vi "CRYGraph Property Window Intensity.vi"(9 "Tab Name":string, 10 "Graph VI Ref":refnum<vi>) -> ()   [LabVIEW 2013]
uses:
  Control/CRYIntensity Property.ctl
panel:
  out "CursorLineStyle":string
  out "CursorLineWidth":string
  out "CursorPointStyle":string
  out "CursorStyle":string
  in  "No Data":bool
  in  "Draw":bool
  in  "Intensity Property":T1 {"Type" items=["Rectangle"=0, "Hanning"=1, "Hamming"=2, "Blackman-Harris"=3, "Exact Blackman"=4, "Blackman"=5, "Flat Top"=6, "4 Term B-Harris"=7, "7 Term B-Harris"=8, "Low Sidelobe"=9, "Blackman Nuttall"=11, "Triangle"=30, "Bartlett-Hanning"=31, "Bohman"=32, "Parzen"=33, "Welch"=34, "Kaiser"=60, "Dolph-Chebyshev"=61, "Gaussian"=62]}
  in  "Intensity Tab":enum32{"Title", "Plot", "Cursor"}(tab)
  in  "Background Color":u32(colorbox) caption="aa"
  in  "Title Name":string caption="aa"
  in  "Length":i32=1 caption="aa" min=1 step=1
  in  "Type":u32(ring) caption="aa" items=["Rectangle"=0, "Hanning"=1, "Hamming"=2, "Blackman-Harris"=3, "Exact Blackman"=4, "Blackman"=5, "Flat Top"=6, "4 Term B-Harris"=7, "7 Term B-Harris"=8, "Low Sidelobe"=9, "Blackman Nuttall"=11, "Triangle"=30, "Bartlett-Hanning"=31, "Bohman"=32, "Parzen"=33, "Welch"=34, "Kaiser"=60, "Dolph-Chebyshev"=61, "Gaussian"=62]
  out "Window":bool caption="aa"
  in  "Frequency Bins":i32=1 caption="aa间隔" min=1 step=1
  in  "Time Steps":i32=1 caption="aa" min=1 step=1
  out "Time-Freq Sampling":bool caption="aa"
  in  "ColorMap Type":u16(ring) caption="aa" items=["Fire", "Rainbow", "Log up", "Log down", "Colour", "Ice"]
  in  "Show Cursors":bool caption="aa"
  in  "Cursor Tab":enum32{"Page 1"}(tab)
  in  "CursorPointStyle16":bool
  in  "CursorPointStyle15":bool
  in  "CursorPointStyle14":bool
  in  "CursorPointStyle13":bool
  in  "CursorPointStyle12":bool
  in  "CursorPointStyle11":bool
  in  "CursorPointStyle10":bool
  in  "CursorPointStyle9":bool
  in  "CursorPointStyle8":bool
  in  "CursorPointStyle7":bool
  in  "CursorPointStyle6":bool
  in  "CursorPointStyle5":bool
  in  "CursorPointStyle4":bool
  in  "CursorPointStyle3":bool
  in  "CursorPointStyle2":bool
  in  "CursorPointStyle1":bool
  in  "CursorPointStyle0":bool
  in  "CursorLineWidth5":bool
  in  "CursorLineWidth1":bool
  in  "CursorLineWidth4":bool
  in  "CursorLineWidth3":bool
  in  "CursorLineWidth2":bool
  in  "CursorLineWidth0":bool
  in  "CursorLineStyle4":bool
  in  "CursorLineStyle3":bool
  in  "CursorLineStyle2":bool
  in  "CursorLineStyle0":bool
  in  "CursorLineStyle1":bool
  in  "Cursor Items":u16(ring)
  in  "CursorStyle8":bool
  in  "CursorStyle4":bool
  in  "CursorStyle5":bool
  in  "CursorStyle7":bool
  in  "CursorStyle6":bool
  in  "CursorStyle3":bool
  in  "CursorStyle2":bool
  in  "CursorStyle1":bool
  in  "CursorStyle0":bool
  in  "Cursor color":u32(colorbox) caption="aa"
  in  "OK":bool
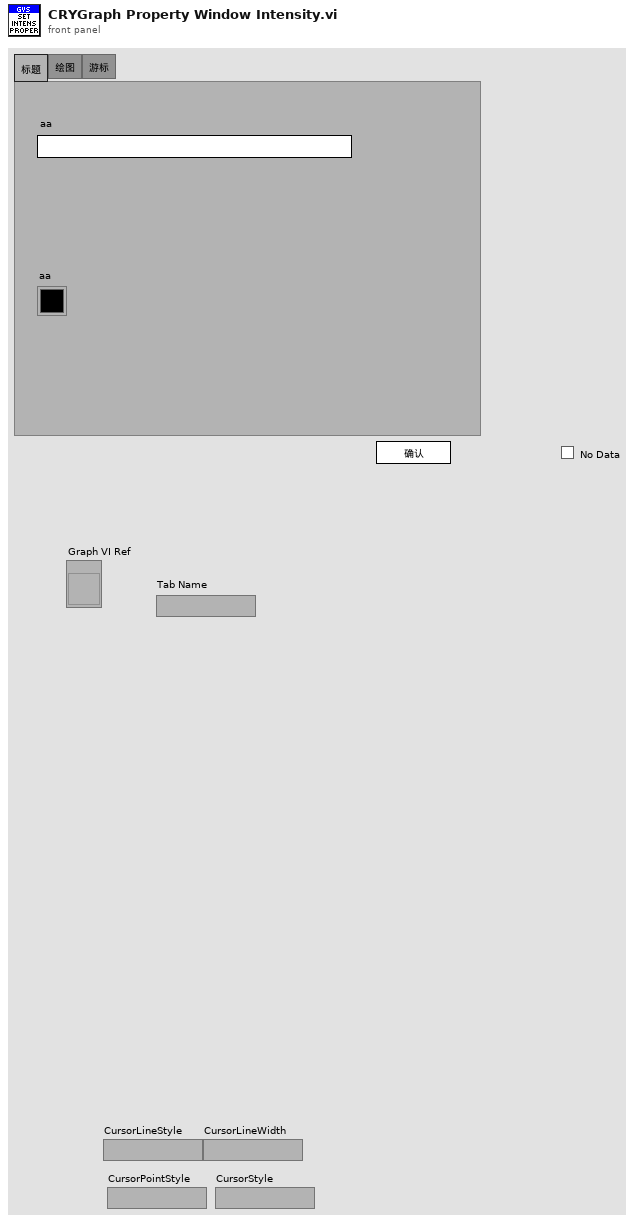
[diagram p1: front panel]
types:
  T1 = typedef "CRYIntensity Property.ctl" = cluster{"Time Steps":i32, "Frequency Bins":i32, "Type":u32, "Length":i32, "Map Type":enum16{"fire", "rainbow", "grey", "inverse grey", "ice", "original"}}
  T2 = enum32{"Page Enabled", "Page Disabled", "Page Disabled & Grayed"}
  T3 = enum16{"fire", "rainbow", "grey", "inverse grey", "ice", "original"}
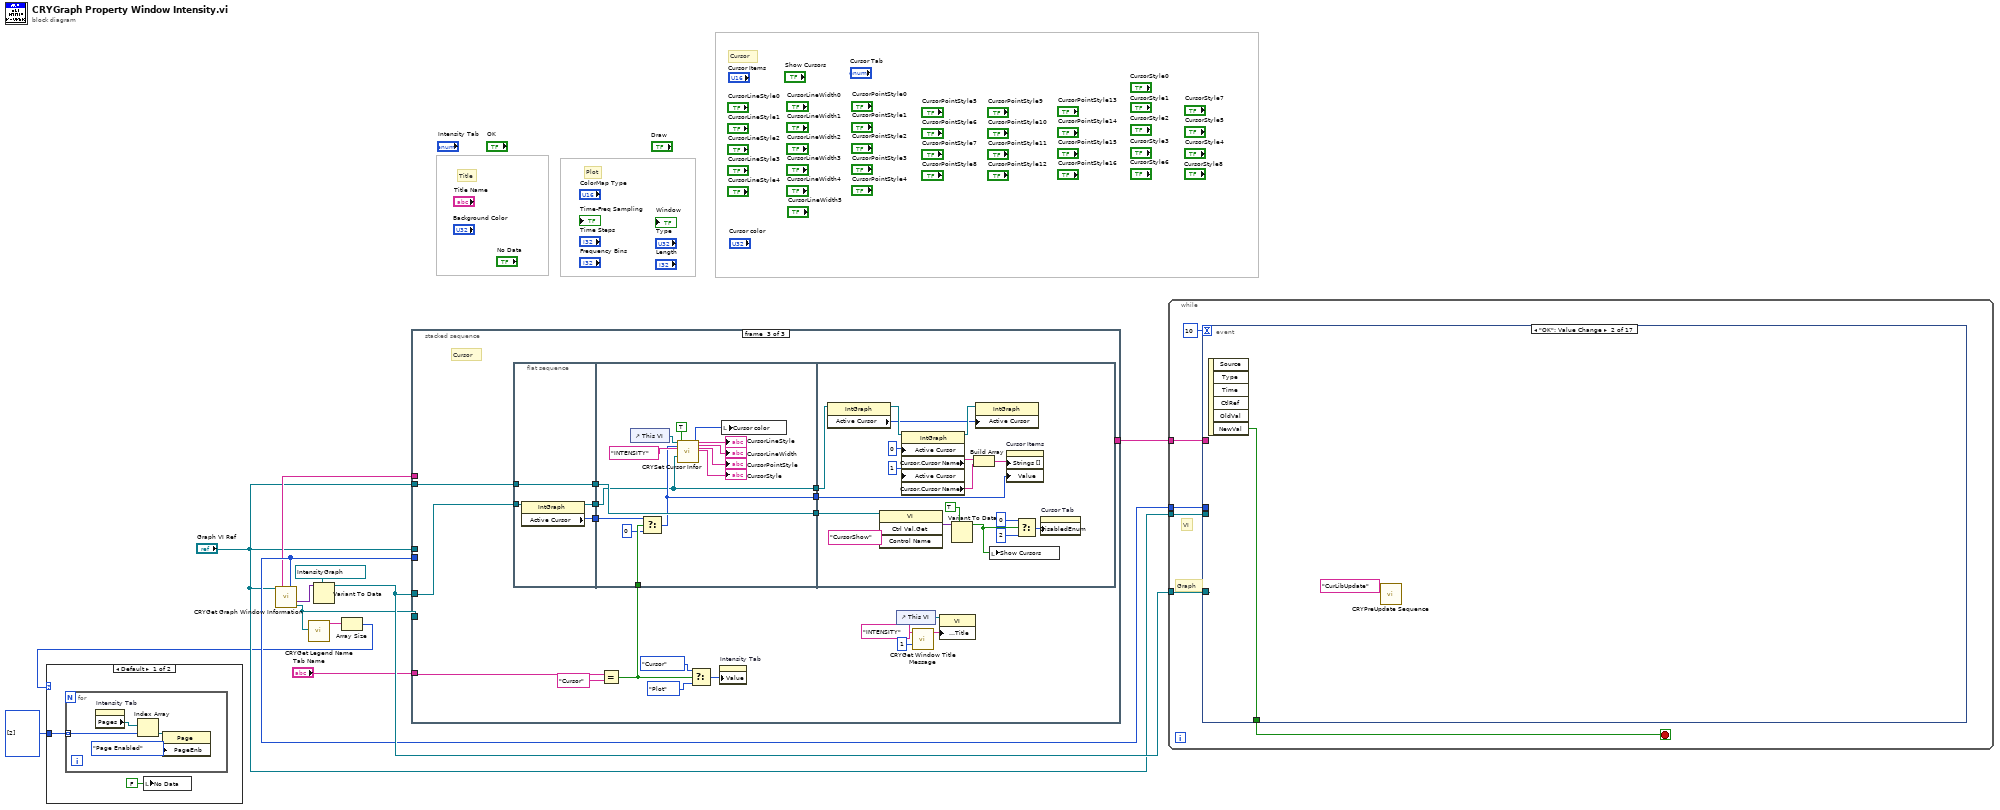
[diagram p0: block diagram]
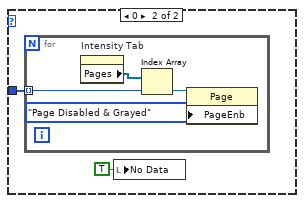
[diagram p2: hidden frame]
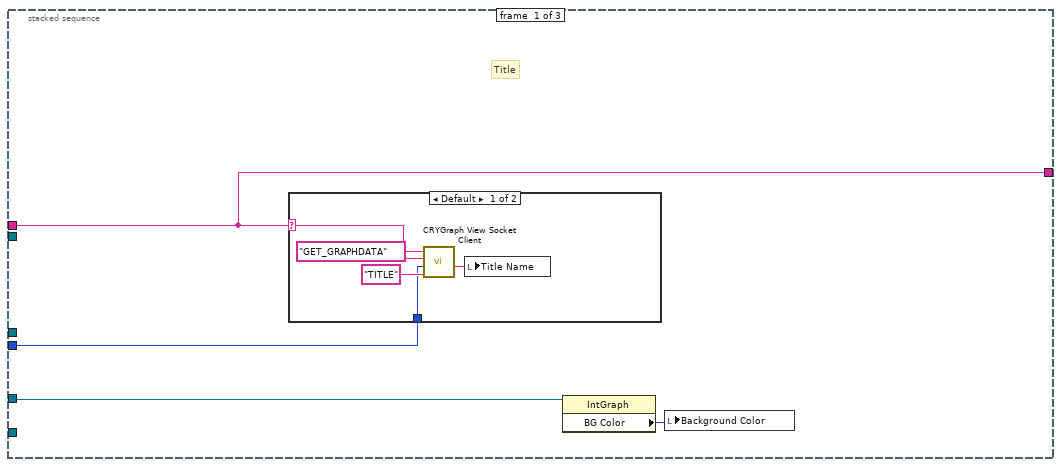
[diagram p3: hidden frame]
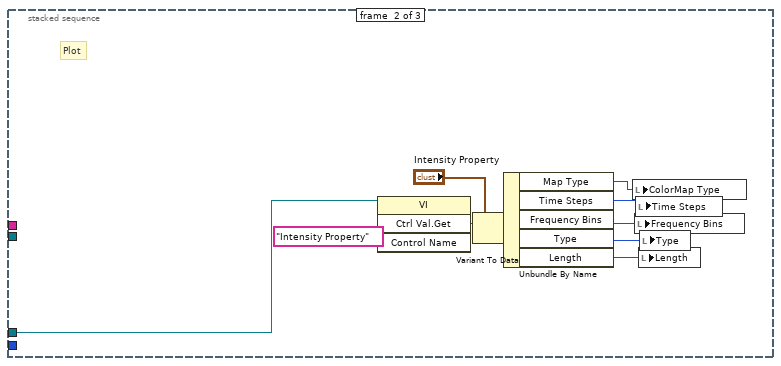
[diagram p5: hidden frame]
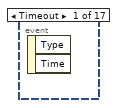
[diagram p6: hidden frame]
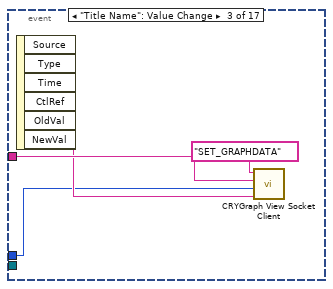
[diagram p7: hidden frame]
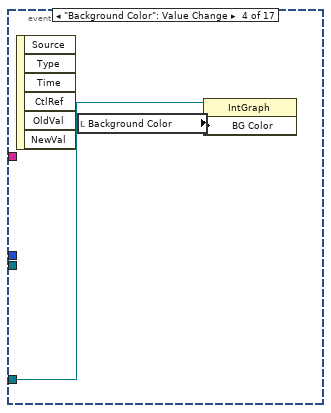
[diagram p8: hidden frame]
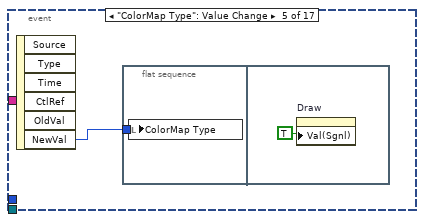
[diagram p9: hidden frame]
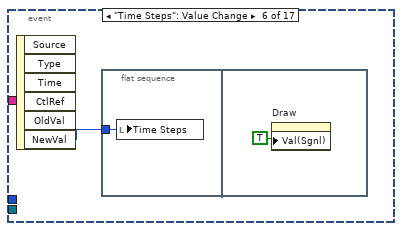
[diagram p10: hidden frame]
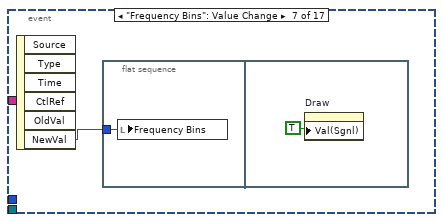
[diagram p11: hidden frame]
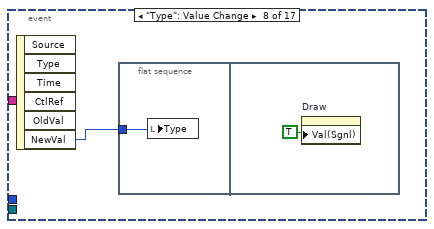
[diagram p12: hidden frame]
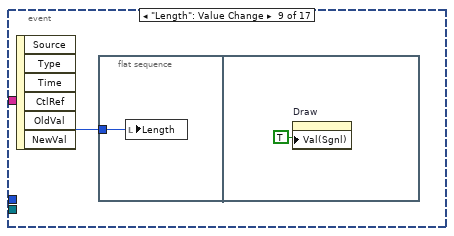
[diagram p13: hidden frame]
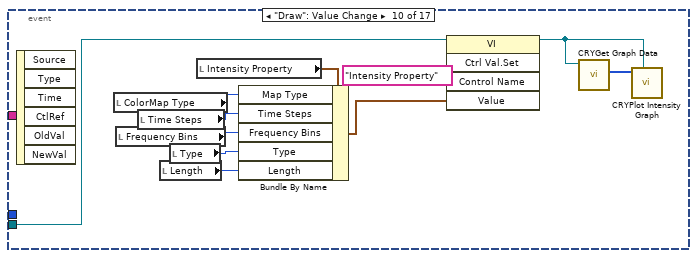
[diagram p14: hidden frame]
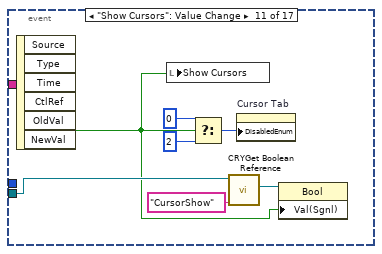
[diagram p15: hidden frame]
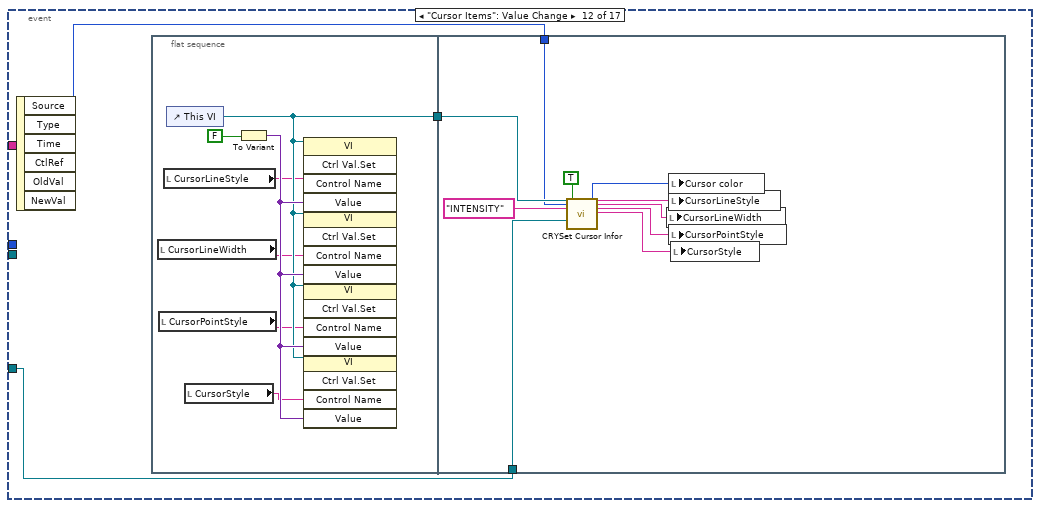
[diagram p16: hidden frame]
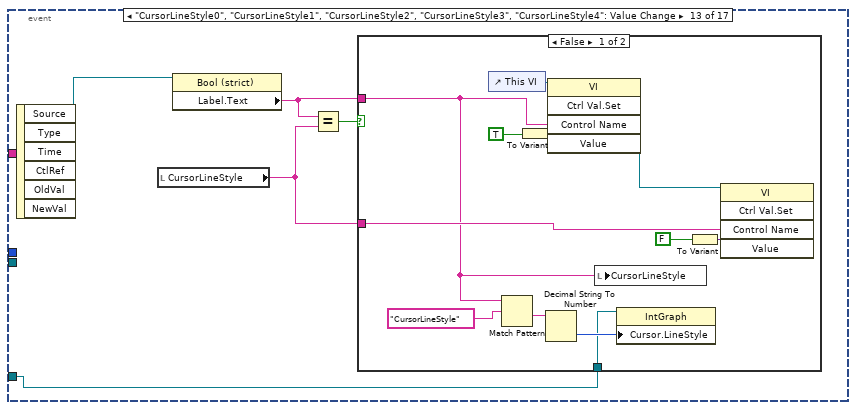
[diagram p17: hidden frame]
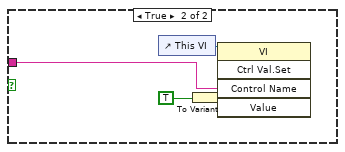
[diagram p18: hidden frame]
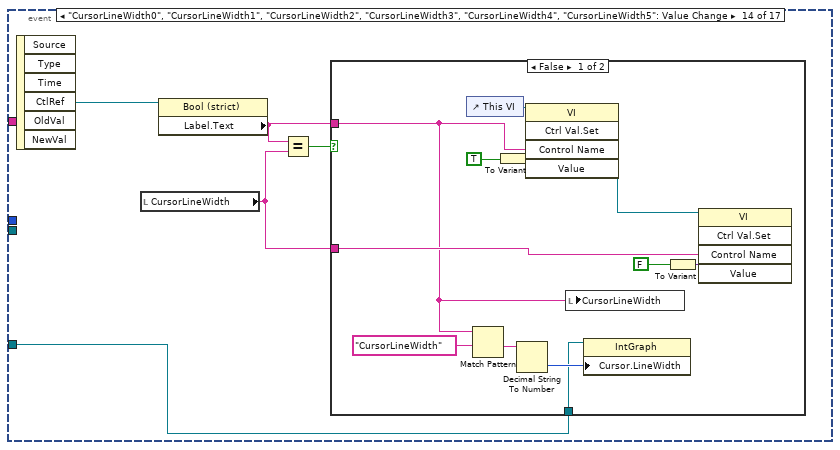
[diagram p19: hidden frame]
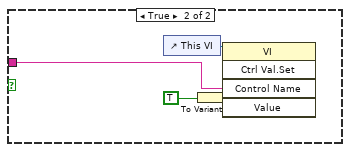
[diagram p20: hidden frame]
diagram:
  # "Cursor"
  # "Title"
  # "Plot"
  n1 = call "CRYGet Graph Window Information.vi"("pGraph VI In"="Graph VI Ref") -> ("Queue Name Out"=w10:string, "Graph Number Out"=w11:i32, "Graph Control Ref Out"=w4:variant, "Legend Ref Out"=w7:refnum<vi>)  [unwired: 4 in, 7 out]
  n2 = call "CRYGet Legend Name.vi"("MCListbox Refnum"=w7) -> ("Names Out"=w2:string[])  [unwired: 1 in, 9 out]
  n3 = Variant To Data(type=refnum<vi> refnum ("Graph Ref"), Variant=w4) -> (data=w12:refnum<vi>)  [unwired: 1 in, 1 out]
  n4 = Array Size(array=w2) -> (size(s)=w1:i32)
  n5 = case shown="Default" w1 {
    tunnel: i32[] [2] -> [w13 w19]
    frame Default {
      n6 = for {
        tunnel: w13 -> [w16] mode=indexing
        n7 = property on="Intensity Tab" class="TabCtl (strict)"() -> ("Pages"=w15:refnum<vi>[])  [unwired: 2 in, 2 out]
        n8 = Index Array(array=w15, index=w16) -> (element=w17:refnum<vi>)
        n9 = property class="Page"(reference=w17, "PageEnb"=T2."Page Enabled" ("Page Enabled State")) -> ()  [unwired: 1 in, 2 out]
      }
      n10 = local write "No Data"(FALSE ("No Data")) -> ()
    }
    frame 0 {
      n11 = for {
        tunnel: w19 -> [w21] mode=indexing
        n12 = property on="Intensity Tab" class="TabCtl (strict)"() -> ("Pages"=w22:refnum<vi>[])  [unwired: 2 in, 2 out]
        n13 = Index Array(array=w22, index=w21) -> (element=w23:refnum<vi>)
        n14 = property class="Page"(reference=w23, "PageEnb"=T2."Page Disabled & Grayed" ("Page Enabled State")) -> ()  [unwired: 1 in, 2 out]
      }
      n15 = local write "No Data"(TRUE ("No Data")) -> ()
    }
  }
  n16 = stacked-sequence {
    tunnel: w12 -> [w27 _ w49]
    tunnel: w11 -> [w26 _ _]
    tunnel: w7 -> [_ _ _]
    tunnel: "Graph VI Ref" -> [_ w41 _]
    tunnel: w10 -> [w25 _ _]
    tunnel: [w25 _ _] -> w9
    tunnel: "Tab Name" -> [_ _ w45]
    tunnel: "Graph VI Ref" -> [_ _ w48]
    frame #0 {
      # "Title"
      n17 = case shown="Default" w25 {
        selector: w25 -> [w30 _]
        tunnel: w26 -> [w31 _]
        frame Default {
          n18 = call "CRYGraph View Socket Client.vi"("sOption"="TITLE", "nData"=w31, "sData"=w30, "sAction"="GET_GRAPHDATA") -> ("sData Out"=w29:string)  [unwired: 4 in, 3 out]
          n19 = local write "Title Name"(w29) -> ()
        }
        frame "test DataView" {
        }
      }
      n20 = property class="IntGraph"(reference=w27) -> ("BG Color"=w28:u32)  [unwired: 1 in, 2 out]
      n21 = local write "Background Color"(w28) -> ()
    }
    frame #1 {
      # "Plot"
      n22 = invoke class="VI" method="Ctrl Val.Get"(reference=w41, "Control Name"="Intensity Property") -> ("Get Control Value Variant"=w42:variant)  [unwired: 2 in, 3 out]
      n23 = Variant To Data(type="Intensity Property", Variant=w42) -> (data=w39:T1)  [unwired: 1 in, 1 out]
      n24 = Unbundle By Name(w39) -> ("Map Type"=w38:T3, "Time Steps"=w37:i32, "Frequency Bins"=w36:i32, "Type"=w35:u32, "Length"=w34:i32)
      n25 = local write "ColorMap Type"(w38) -> ()
      n26 = local write "Frequency Bins"(w36) -> ()
      n27 = local write "Time Steps"(w37) -> ()
      n28 = local write "Length"(w34) -> ()
      n29 = local write "Type"(w35) -> ()
    }
    frame #2 {
      # "Cursor"
      n30 = flat-sequence {
        tunnel: w48 -> [w65]
        tunnel: w49 -> [w64]
        tunnel: [w63] -> w61
        tunnel: [w65] -> w60
        tunnel: [w62] -> w59
        tunnel: [w66] -> w58
        tunnel: [w71] -> w57
        tunnel: w61 -> [w66]
        tunnel: w60 -> [w71]
        tunnel: w51 -> [w70]
        tunnel: w59 -> [w68]
        tunnel: [w67] -> w56
        tunnel: w58 -> [w84]
        tunnel: w57 -> [w85]
        tunnel: w56 -> [w80]
        frame #0 {
          n31 = property class="IntGraph"(reference=w64) -> (reference out=w63:refnum<vi>, "Active Cursor"=w62:u32)  [unwired: 1 in, 1 out]
        }
        frame #1 {
          n32 = control-ref of="This VI"() -> (w72:refnum<vi>)
          n33 = Select(t=w68, s=w70, f=u32 0 ("Active Cursor")) -> (s? t:f=w67:u32)
          n34 = call "CRYSet Cursor Infor.vi"("This VI"=w72, "Active Cursor"=w67, "Graph Type"="INTENSITY", "Intensity Graph Ref"=w66, "Property Set?"=TRUE) -> ("Cursor Color"=w79:u32, "CursorLineStyle"=→"CursorLineStyle":string, "CursorLineWidth"=→"CursorLineWidth":string, "CursorPointStyle"=→"CursorPointStyle":string, "CursorStyle"=→"CursorStyle":string)  [unwired: 17 in, 1 out]
          n35 = local write "Cursor color"(w79) -> ()
        }
        frame #2 {
          n36 = property class="IntGraph"(reference=w84) -> (reference out=w83:refnum<vi>, "Active Cursor"=w81:u32)  [unwired: 1 in, 1 out]
          n37 = invoke class="VI" method="Ctrl Val.Get"(reference=w85, "Control Name"="CursorShow") -> ("Get Control Value Variant"=w90:variant)  [unwired: 2 in, 3 out]
          n38 = property class="IntGraph"(reference=w83, "Active Cursor"=u32 0, "Active Cursor"=u32 1) -> (reference out=w82:refnum<vi>, "Cursor.Cursor Name"=w95:string, "Cursor.Cursor Name"=w94:string)  [unwired: 1 in, 1 out]
          n39 = Variant To Data(type=TRUE ("Visible"), Variant=w90) -> (data=w92:bool)  [unwired: 1 in, 1 out]
          n40 = Build Array(w95, w94) -> (w93:string[])
          n41 = property class="IntGraph"(reference=w82, "Active Cursor"=w81) -> ()  [unwired: 1 in, 2 out]
          n42 = local write "Show Cursors"(w92) -> ()
          n43 = property on="Cursor Items" class="Ring (strict)"("Strings []"=w93, "Value"=w80) -> ()  [unwired: 2 in, 2 out]
          n44 = Select(t=0, s=w92, f=2) -> (s? t:f=w88:i32)
          n45 = property on="Cursor Tab" class="TabCtl (strict)"("DisabledEnum"=w88) -> ()  [unwired: 2 in, 2 out]
        }
      }
      n46 = Equal?(x=w45, y="Cursor" ("Graph Type")) -> (x = y?=w51:bool)
      n47 = Select(t=enum32{"Title", "Plot", "Cursor"}."Cursor" ("Intensity Tab"), s=w51, f=enum32{"Title", "Plot", "Cursor"}."Plot" ("Intensity Tab")) -> (s? t:f=w46:enum32{"Title", "Plot", "Cursor"})
      n48 = property on="Intensity Tab" class="TabCtl (strict)"("Value"=w46) -> ()  [unwired: 2 in, 2 out]
      n49 = control-ref of="This VI"() -> (w55:refnum<vi>)
      n50 = call "CRYGet Window Title Message.vi"("No"=1 ("Error No"), "Kind"="INTENSITY") -> ("Multibyte String"=w54:string)  [unwired: 4 in, 5 out]
      n51 = property class="VI"(reference=w55, "Front Panel.Title"=w54) -> ()  [unwired: 1 in, 2 out]
    }
  }
  n52 = while {
    tunnel: w12 -> [w102]
    tunnel: w11 -> [w101]
    tunnel: "Graph VI Ref" -> [w100]
    tunnel: w9 -> [w99]
    stop <- w103 stop-if-true
    # "Graph"
    # "VI"
    n53 = event shown="[1] \"OK\": Value Change" {
      selector: _ -> [_ _ _ _ _ _ _ _ _ _ _ _ _ _ _ _ _]
      dyn-events: _ -> [_ _ _ _ _ _ _ _ _ _ _ _ _ _ _ _ _]
      timeout: 10 -> [_ _ _ _ _ _ _ _ _ _ _ _ _ _ _ _ _]
      tunnel: [_ w105 _ _ _ _ _ _ _ _ _ _ _ _ _ _ _] -> w103
      tunnel: w102 -> [_ _ _ w111 _ _ _ _ _ _ _ w146 w166 w186 w207 w228 w250]
      tunnel: w101 -> [_ _ w106 _ _ _ _ _ _ _ _ _ _ _ _ _ _]
      tunnel: w100 -> [_ _ _ _ _ _ _ _ _ w137 w139 _ _ _ _ _ w249]
      tunnel: w99 -> [_ _ w108 _ _ _ _ _ _ _ _ _ _ _ _ _ _]
      event Timeout {
        n54 = event-data() -> ()  [unwired: 3 out]
      }
      event "OK": Value Change {
        n55 = event-data() -> ("NewVal"=w105:bool)  [unwired: 6 out]
        n56 = call "CRYPreUpdate Sequence.vi"("EventName"="CurLibUpdate") -> ()  [unwired: 15 in]
      }
      event "Title Name": Value Change {
        n57 = event-data() -> ("NewVal"=w107:string)  [unwired: 6 out]
        n58 = call "CRYGraph View Socket Client.vi"("sOption"=w107, "nData"=w106, "sData"=w108, "sAction"="SET_GRAPHDATA") -> ()  [unwired: 4 in, 4 out]
      }
      event "Background Color": Value Change {
        n59 = event-data() -> ()  [unwired: 7 out]
        n60 = local read "Background Color"() -> (w110:u32)
        n61 = property class="IntGraph"(reference=w111, "BG Color"=w110) -> ()  [unwired: 1 in, 2 out]
      }
      event "ColorMap Type": Value Change {
        n62 = event-data() -> ("NewVal"=w112:u16)  [unwired: 6 out]
        n63 = flat-sequence {
          tunnel: w112 -> [w113]
          frame #0 {
            n64 = local write "ColorMap Type"(w113) -> ()
          }
          frame #1 {
            n65 = property on="Draw" class="Bool (strict)"("Val(Sgnl)"=TRUE ("Value (Signaling)")) -> ()  [unwired: 2 in, 2 out]
          }
        }
      }
      event "Time Steps": Value Change {
        n66 = event-data() -> ("NewVal"=w115:i32)  [unwired: 6 out]
        n67 = flat-sequence {
          tunnel: w115 -> [w116]
          frame #0 {
            n68 = local write "Time Steps"(w116) -> ()
          }
          frame #1 {
            n69 = property on="Draw" class="Bool (strict)"("Val(Sgnl)"=TRUE ("Value (Signaling)")) -> ()  [unwired: 2 in, 2 out]
          }
        }
      }
      event "Frequency Bins": Value Change {
        n70 = event-data() -> ("NewVal"=w118:i32)  [unwired: 6 out]
        n71 = flat-sequence {
          tunnel: w118 -> [w119]
          frame #0 {
            n72 = local write "Frequency Bins"(w119) -> ()
          }
          frame #1 {
            n73 = property on="Draw" class="Bool (strict)"("Val(Sgnl)"=TRUE ("Value (Signaling)")) -> ()  [unwired: 2 in, 2 out]
          }
        }
      }
      event "Type": Value Change {
        n74 = event-data() -> ("NewVal"=w121:u32)  [unwired: 6 out]
        n75 = flat-sequence {
          tunnel: w121 -> [w122]
          frame #0 {
            n76 = local write "Type"(w122) -> ()
          }
          frame #1 {
            n77 = property on="Draw" class="Bool (strict)"("Val(Sgnl)"=TRUE ("Value (Signaling)")) -> ()  [unwired: 2 in, 2 out]
          }
        }
      }
      event "Length": Value Change {
        n78 = event-data() -> ("NewVal"=w124:i32)  [unwired: 6 out]
        n79 = flat-sequence {
          tunnel: w124 -> [w125]
          frame #0 {
            n80 = local write "Length"(w125) -> ()
          }
          frame #1 {
            n81 = property on="Draw" class="Bool (strict)"("Val(Sgnl)"=TRUE ("Value (Signaling)")) -> ()  [unwired: 2 in, 2 out]
          }
        }
      }
      event "Draw": Value Change {
        n82 = event-data() -> ()  [unwired: 7 out]
        n83 = local read "ColorMap Type"() -> (w134:u16)
        n84 = local read "Frequency Bins"() -> (w132:i32)
        n85 = local read "Time Steps"() -> (w133:i32)
        n86 = local read "Length"() -> (w130:i32)
        n87 = local read "Type"() -> (w131:u32)
        n88 = local read "Intensity Property"() -> (w135:T1)
        n89 = Bundle By Name(cluster=w135, "Map Type"=w134, "Time Steps"=w133, "Frequency Bins"=w132, "Type"=w131, "Length"=w130) -> (w129:T1)
        n90 = invoke class="VI" method="Ctrl Val.Set"(reference=w137, "Control Name"="Intensity Property", "Value"=w129) -> (reference out=w127:refnum<vi>)  [unwired: 2 in, 4 out]
        n91 = call "CRYGet Graph Data.vi"("pGraph VI"=w127) -> ("Rows"=w128:i32[])  [unwired: 2 in, 8 out]
        n92 = call "CRYPlot Intensity Graph.vi"("pGraph VI In"=w127, "Selected Rows In"=w128) -> ()  [unwired: 6 in, 4 out]
      }
      event "Show Cursors": Value Change {
        n93 = event-data() -> ("NewVal"=w138:bool)  [unwired: 6 out]
        n94 = local write "Show Cursors"(w138) -> ()
        n95 = Select(t=0, s=w138, f=2) -> (s? t:f=w140:i32)
        n96 = call "CRYGet Boolean Reference.vi"("Label Name"="CursorShow", "VI Refnum"=w139) -> ("Boolean Ref"=w144:refnum<vi>)  [unwired: 7 in, 2 out]
        n97 = property on="Cursor Tab" class="TabCtl (strict)"("DisabledEnum"=w140) -> ()  [unwired: 2 in, 2 out]
        n98 = property class="Bool"(reference=w144, "Val(Sgnl)"=w138) -> ()  [unwired: 1 in, 2 out]
      }
      event "Cursor Items": Value Change {
        n99 = event-data() -> ("NewVal"=w145:u16)  [unwired: 6 out]
        n100 = flat-sequence {
          tunnel: [w152] -> w147
          tunnel: w147 -> [w157]
          tunnel: w145 -> [w156]
          tunnel: w146 -> [w155]
          frame #0 {
            n101 = local read "CursorLineWidth"() -> (w150:string)
            n102 = local read "CursorPointStyle"() -> (w149:string)
            n103 = local read "CursorLineStyle"() -> (w151:string)
            n104 = control-ref of="This VI"() -> (w152:refnum<vi>)
            n105 = local read "CursorStyle"() -> (w148:string)
            n106 = To Variant(anything=FALSE) -> (Variant=w154:variant)
            n107 = invoke class="VI" method="Ctrl Val.Set"(reference=w152, "Control Name"=w151, "Value"=w154) -> ()  [unwired: 2 in, 5 out]
            n108 = invoke class="VI" method="Ctrl Val.Set"(reference=w152, "Control Name"=w150, "Value"=w154) -> ()  [unwired: 2 in, 5 out]
            n109 = invoke class="VI" method="Ctrl Val.Set"(reference=w152, "Control Name"=w149, "Value"=w154) -> ()  [unwired: 2 in, 5 out]
            n110 = invoke class="VI" method="Ctrl Val.Set"(reference=w152, "Control Name"=w148, "Value"=w154) -> ()  [unwired: 2 in, 5 out]
          }
          frame #1 {
            n111 = call "CRYSet Cursor Infor.vi"("This VI"=w157, "Active Cursor"=w156, "Graph Type"="INTENSITY", "Intensity Graph Ref"=w155, "Property Set?"=TRUE) -> ("Cursor Color"=w158:u32, "CursorLineStyle"=w161:string, "CursorLineWidth"=w162:string, "CursorPointStyle"=w163:string, "CursorStyle"=w164:string)  [unwired: 17 in, 1 out]
            n112 = local write "CursorLineWidth"(w162) -> ()
            n113 = local write "Cursor color"(w158) -> ()
            n114 = local write "CursorLineStyle"(w161) -> ()
            n115 = local write "CursorPointStyle"(w163) -> ()
            n116 = local write "CursorStyle"(w164) -> ()
          }
        }
      }
      event "CursorLineStyle0", "CursorLineStyle1", "CursorLineStyle2", "CursorLineStyle3", "CursorLineStyle4": Value Change {
        n117 = event-data() -> ("CtlRef"=w165:refnum<vi>)  [unwired: 6 out]
        n118 = local read "CursorLineStyle"() -> (w169:string)
        n119 = property class="Bool (strict)"(reference=w165) -> ("Label.Text"=w167:string)  [unwired: 1 in, 2 out]
        n120 = Equal?(x=w167, y=w169) -> (x = y?=w168:bool)
        n121 = case shown="False" w168 {
          tunnel: w167 -> [w170 w182]
          tunnel: w169 -> [w180 _]
          tunnel: w166 -> [w171 _]
          frame False {
            n122 = control-ref of="This VI"() -> (w181:refnum<vi>)
            n123 = Match Pattern(string=w170, regular expression="CursorLineStyle") -> (after substring=w173:string)  [unwired: 4 out]
            n124 = To Variant(anything=TRUE) -> (Variant=w178:variant)
            n125 = Decimal String To Number(string=w173) -> (number=w172:i32)  [unwired: 3 out]
            n126 = invoke class="VI" method="Ctrl Val.Set"(reference=w181, "Control Name"=w170, "Value"=w178) -> (reference out=w179:refnum<vi>)  [unwired: 2 in, 4 out]
            n127 = local write "CursorLineStyle"(w170) -> ()
            n128 = property class="IntGraph"(reference=w171, "Cursor.LineStyle"=w172) -> ()  [unwired: 1 in, 2 out]
            n129 = To Variant(anything=FALSE) -> (Variant=w176:variant)
            n130 = invoke class="VI" method="Ctrl Val.Set"(reference=w179, "Control Name"=w180, "Value"=w176) -> ()  [unwired: 2 in, 5 out]
          }
          frame True {
            n131 = control-ref of="This VI"() -> (w185:refnum<vi>)
            n132 = To Variant(anything=TRUE) -> (Variant=w184:variant)
            n133 = invoke class="VI" method="Ctrl Val.Set"(reference=w185, "Control Name"=w182, "Value"=w184) -> ()  [unwired: 2 in, 5 out]
          }
        }
      }
      event "CursorLineWidth0", "CursorLineWidth1", "CursorLineWidth2", "CursorLineWidth3", "CursorLineWidth4", "CursorLineWidth5": Value Change {
        n134 = event-data() -> ("CtlRef"=w187:refnum<vi>)  [unwired: 6 out]
        n135 = local read "CursorLineWidth"() -> (w190:string)
        n136 = property class="Bool (strict)"(reference=w187) -> ("Label.Text"=w188:string)  [unwired: 1 in, 2 out]
        n137 = Equal?(x=w188, y=w190) -> (x = y?=w189:bool)
        n138 = case shown="False" w189 {
          tunnel: w188 -> [w191 w203]
          tunnel: w190 -> [w201 _]
          tunnel: w186 -> [w192 _]
          frame False {
            n139 = control-ref of="This VI"() -> (w202:refnum<vi>)
            n140 = Match Pattern(string=w191, regular expression="CursorLineWidth") -> (after substring=w194:string)  [unwired: 4 out]
            n141 = To Variant(anything=TRUE) -> (Variant=w199:variant)
            n142 = Decimal String To Number(string=w194) -> (number=w195:i32)  [unwired: 3 out]
            n143 = invoke class="VI" method="Ctrl Val.Set"(reference=w202, "Control Name"=w191, "Value"=w199) -> (reference out=w200:refnum<vi>)  [unwired: 2 in, 4 out]
            n144 = local write "CursorLineWidth"(w191) -> ()
            n145 = property class="IntGraph"(reference=w192, "Cursor.LineWidth"=w195) -> ()  [unwired: 1 in, 2 out]
            n146 = To Variant(anything=FALSE) -> (Variant=w197:variant)
            n147 = invoke class="VI" method="Ctrl Val.Set"(reference=w200, "Control Name"=w201, "Value"=w197) -> ()  [unwired: 2 in, 5 out]
          }
          frame True {
            n148 = control-ref of="This VI"() -> (w206:refnum<vi>)
            n149 = To Variant(anything=TRUE) -> (Variant=w205:variant)
            n150 = invoke class="VI" method="Ctrl Val.Set"(reference=w206, "Control Name"=w203, "Value"=w205) -> ()  [unwired: 2 in, 5 out]
          }
        }
      }
      event "CursorPointStyle0", "CursorPointStyle1", "CursorPointStyle2", "CursorPointStyle3", "CursorPointStyle4", "CursorPointStyle5", "CursorPointStyle6", "CursorPointStyle7", "CursorPointStyle8", "CursorPointStyle9", "CursorPointStyle10", "CursorPointStyle11", "CursorPointStyle12", "CursorPointStyle13", "CursorPointStyle14", "CursorPointStyle15", "CursorPointStyle16": Value Change {
        n151 = event-data() -> ("CtlRef"=w208:refnum<vi>)  [unwired: 6 out]
        n152 = local read "CursorPointStyle"() -> (w211:string)
        n153 = property class="Bool (strict)"(reference=w208) -> ("Label.Text"=w209:string)  [unwired: 1 in, 2 out]
        n154 = Equal?(x=w209, y=w211) -> (x = y?=w210:bool)
        n155 = case shown="False" w210 {
          tunnel: w209 -> [w212 w224]
          tunnel: w211 -> [w222 _]
          tunnel: w207 -> [w213 _]
          frame False {
            n156 = control-ref of="This VI"() -> (w223:refnum<vi>)
            n157 = To Variant(anything=TRUE) -> (Variant=w220:variant)
            n158 = Match Pattern(string=w212, regular expression="CursorPointStyle") -> (after substring=w215:string)  [unwired: 4 out]
            n159 = invoke class="VI" method="Ctrl Val.Set"(reference=w223, "Control Name"=w212, "Value"=w220) -> (reference out=w221:refnum<vi>)  [unwired: 2 in, 4 out]
            n160 = Decimal String To Number(string=w215) -> (number=w216:i32)  [unwired: 3 out]
            n161 = local write "CursorPointStyle"(w212) -> ()
            n162 = property class="IntGraph"(reference=w213, "Cursor.Cursor Point Style"=w216) -> ()  [unwired: 1 in, 2 out]
            n163 = To Variant(anything=FALSE) -> (Variant=w218:variant)
            n164 = invoke class="VI" method="Ctrl Val.Set"(reference=w221, "Control Name"=w222, "Value"=w218) -> ()  [unwired: 2 in, 5 out]
          }
          frame True {
            n165 = control-ref of="This VI"() -> (w227:refnum<vi>)
            n166 = To Variant(anything=TRUE) -> (Variant=w226:variant)
            n167 = invoke class="VI" method="Ctrl Val.Set"(reference=w227, "Control Name"=w224, "Value"=w226) -> ()  [unwired: 2 in, 5 out]
          }
        }
      }
      event "CursorStyle0", "CursorStyle1", "CursorStyle2", "CursorStyle3", "CursorStyle4", "CursorStyle5", "CursorStyle6", "CursorStyle7", "CursorStyle8": Value Change {
        n168 = event-data() -> ("CtlRef"=w229:refnum<vi>)  [unwired: 6 out]
        n169 = local read "CursorStyle"() -> (w232:string)
        n170 = property class="Bool (strict)"(reference=w229) -> ("Label.Text"=w230:string)  [unwired: 1 in, 2 out]
        n171 = Equal?(x=w230, y=w232) -> (x = y?=w231:bool)
        n172 = case shown="False" w231 {
          tunnel: w230 -> [w233 w245]
          tunnel: w232 -> [w243 _]
          tunnel: w228 -> [w234 _]
          frame False {
            n173 = control-ref of="This VI"() -> (w244:refnum<vi>)
            n174 = To Variant(anything=TRUE) -> (Variant=w241:variant)
            n175 = Match Pattern(string=w233, regular expression="CursorStyle") -> (after substring=w236:string)  [unwired: 4 out]
            n176 = invoke class="VI" method="Ctrl Val.Set"(reference=w244, "Control Name"=w233, "Value"=w241) -> (reference out=w242:refnum<vi>)  [unwired: 2 in, 4 out]
            n177 = Decimal String To Number(string=w236) -> (number=w237:i32)  [unwired: 3 out]
            n178 = local write "CursorStyle"(w233) -> ()
            n179 = property class="IntGraph"(reference=w234, "Cursor.Cursor Style"=w237) -> ()  [unwired: 1 in, 2 out]
            n180 = To Variant(anything=FALSE) -> (Variant=w239:variant)
            n181 = invoke class="VI" method="Ctrl Val.Set"(reference=w242, "Control Name"=w243, "Value"=w239) -> ()  [unwired: 2 in, 5 out]
          }
          frame True {
            n182 = control-ref of="This VI"() -> (w248:refnum<vi>)
            n183 = To Variant(anything=TRUE) -> (Variant=w247:variant)
            n184 = invoke class="VI" method="Ctrl Val.Set"(reference=w248, "Control Name"=w245, "Value"=w247) -> ()  [unwired: 2 in, 5 out]
          }
        }
      }
      event "Cursor color": Value Change {
        n185 = event-data() -> ("NewVal"=w251:u32)  [unwired: 6 out]
        n186 = property class="IntGraph"(reference=w250) -> (reference out=w253:refnum<vi>, "Active Cursor"=w255:u32)  [unwired: 1 in, 1 out]
        n187 = local read "Cursor Items"() -> (w252:u16)
        n188 = local write "Cursor color"(w251) -> ()
        n189 = property class="IntGraph"(reference=w253, "Active Cursor"=w252, "Cursor.Cursor Color"=w251) -> (reference out=w254:refnum<vi>)  [unwired: 1 in, 1 out]
        n190 = property class="IntGraph"(reference=w254, "Active Cursor"=w255) -> (reference out=w256:refnum<vi>)  [unwired: 1 in, 1 out]
        n191 = flat-sequence {
          tunnel: w249 -> [w257]
          tunnel: w256 -> [_]
          frame #0 {
            n192 = call "CRYGet Boolean Reference.vi"("Label Name"="CursorColor" ("Control Name"), "VI Refnum"=w257) -> ("Boolean Ref"=w259:refnum<vi>)  [unwired: 7 in, 2 out]
            n193 = property class="Bool"(reference=w259, "Val(Sgnl)"=TRUE ("Visible")) -> ()  [unwired: 1 in, 2 out]
          }
        }
      }
    }
  }
